vi "Error.vi"(6 "Abort if errors":bool, 8 "error in (no error)":errorcluster, 10 "Process Error":errorcluster, 11 "Bar in":refnum<class "Bar.lvclass">) -> (0 "error out":errorcluster, 3 "Bar out":refnum<class "Bar.lvclass">)   [LabVIEW 2015, in "Simple Progress Bar.lvlib" / "Bar.lvclass"]
doc: "Display errors & warning from <b>Process Error</b> parameter in the progress bar user interface. If <b>Abort if errors</b> is enabled, any error will abort the process."
uses:
  Bar.lvclass
  Bar.lvclass/Bar.ctl
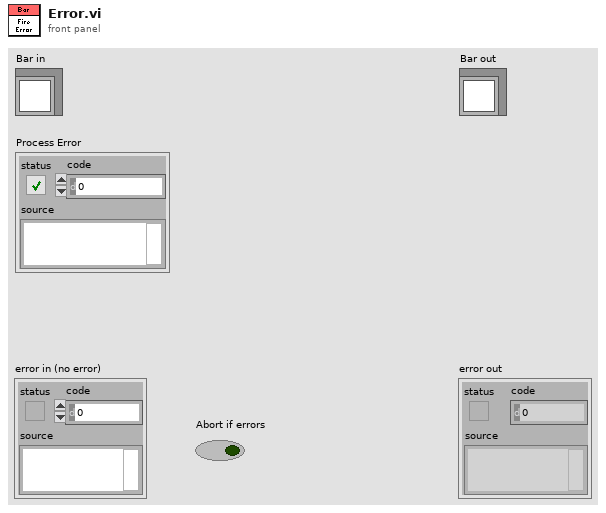
[diagram p1: front panel]
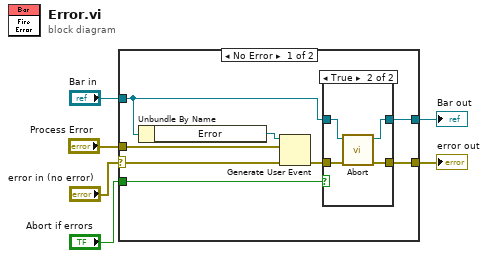
[diagram p0: block diagram]
diagram:
  n1 = case shown="No Error" "error in (no error)" {
    selector: "error in (no error)" -> [w12 w22]
    tunnel: [w11 w22] -> w5
    tunnel: [w9 w21] -> w3
    tunnel: "Bar in" -> [w10 w21]
    tunnel: "Process Error" -> [w8 _]
    tunnel: "Abort if errors" -> [w7 _]
    frame No Error {
      n2 = Unbundle By Name(w10) -> ("Error"=w14:refnum<user-event>)
      n3 = Generate User Event(user event=w14, event data cluster=w8, error in=w12) -> (error out=w13:errorcluster)  [unwired: 1 in, 1 out]
      n4 = case shown="True" w7 {
        tunnel: w10 -> [w16 w17]
        tunnel: w13 -> [w15 w20]
        tunnel: [w15 w19] -> w11
        tunnel: [w16 w18] -> w9
        frame False {
        }
        frame True {
          n5 = call "Abort.vi"("error in (no error)"=w20, "Bar in"=w17) -> ("error out"=w19:errorcluster, "Bar out"=w18:refnum<class "Bar.lvclass">)  [unwired: 8 in]
        }
      }
    }
    frame Error {
    }
  }
  "error out" <- w5
  "Bar out" <- w3
